vi "GDSString_XmlEnumToStringValue.vi"(0 "XmlEnumStringIn":string, 1 "EnumVariantIn(used if String is Empty)":variant, 5 "error in (no error)":errorcluster) -> (14 "EnumValueOut(string)":string, 15 "EnumItems(string)":string[](array[string]), 16 "EnumValueOut(uint16)":u16, 19 "error out":errorcluster)   [LabVIEW 2020]
doc: "Uses a flatten XML string of a Enum-type <B>\"XmlEnumStringIn\"</B> to find the acctually value of the enum.\nThis is normally used when a Enum has been flatten to a variant.\nIt could also take the enum variant as an input\nIt the Variant ENUM is of string type it will send it through without any errors"
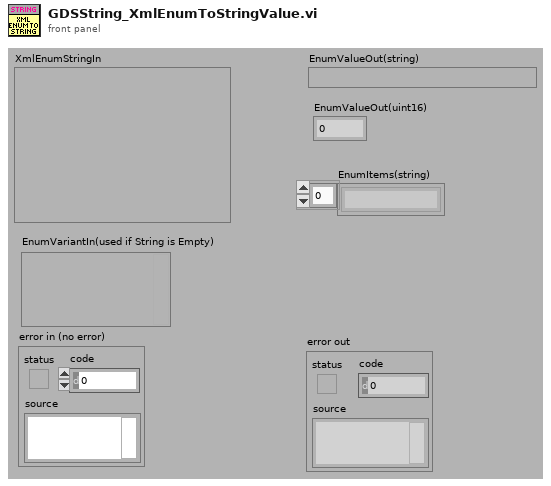
[diagram p1: front panel]
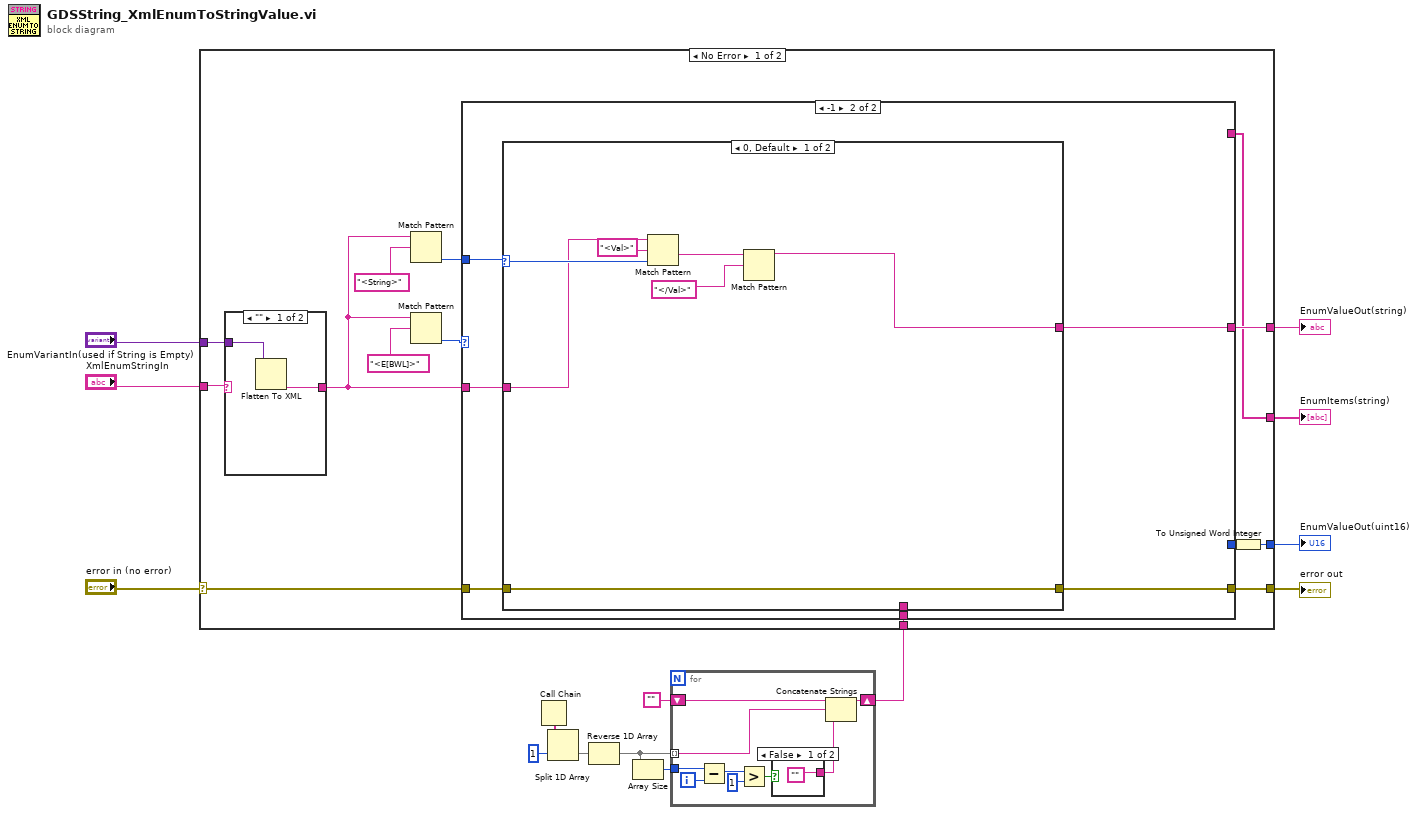
[diagram p0: block diagram]
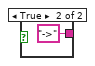
[diagram p2: hidden frame]
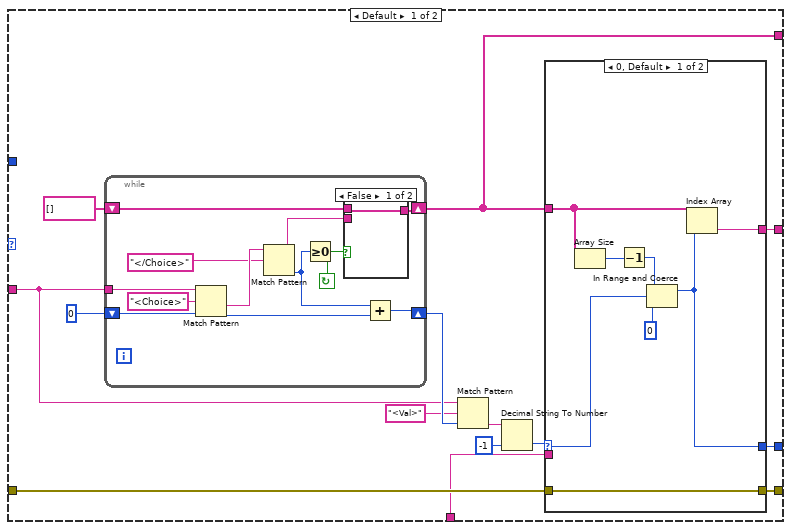
[diagram p4: hidden frame]
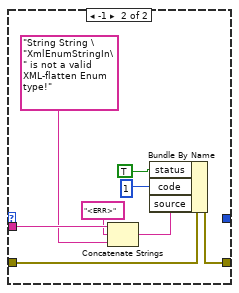
[diagram p5: hidden frame]
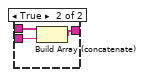
[diagram p6: hidden frame]
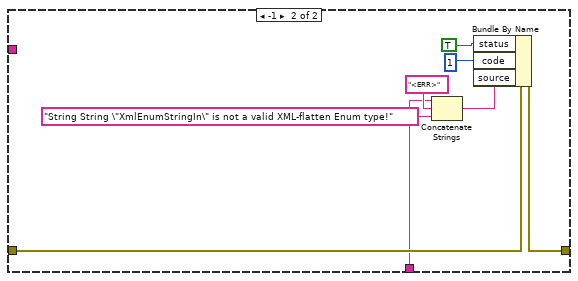
[diagram p7: hidden frame]
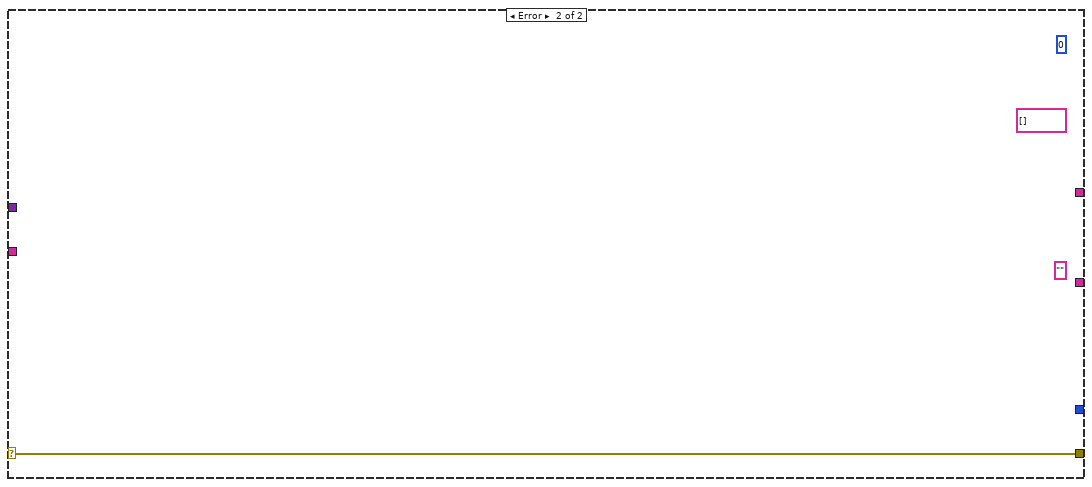
[diagram p8: hidden frame]
diagram:
  n1 = Call Chain() -> (call chain=w2:string[])
  n2 = Split 1D Array(array=w2, index=1) -> (second subarray=w4:string[])  [unwired: 1 out]
  n3 = Reverse 1D Array(array=w4) -> (reversed array=w7:string[])
  n4 = Array Size(array=w7) -> (size(s)=w5:i32)
  n5 = for {
    shift-right: [w15] -> w1
    shift-left: "" -> [w18]
    tunnel: w7 -> [w16] mode=indexing
    tunnel: w5 -> [w23]
    i -> [w22]
    n6 = Subtract(x=w23, y=w22) -> (x-y=w21:i32)
    n7 = Greater?(x=w21, y=1) -> (0:w19:bool)
    n8 = case shown="False" w19 {
      tunnel: ["" "->"] -> w17
      frame False {
      }
      frame True {
      }
    }
    n9 = Concatenate Strings(w18, w16, w17) -> (w15:string)
  }
  n10 = case shown="No Error" "error in (no error)" {
    selector: "error in (no error)" -> [w37 w110]
    tunnel: [w36 w110] -> w13
    tunnel: "XmlEnumStringIn" -> [w32 _]
    tunnel: [w35 _] -> w11
    tunnel: [w33 _] -> w10
    tunnel: "EnumVariantIn(used if String is Empty)" -> [w31 _]
    tunnel: [w27 _] -> w8
    tunnel: w1 -> [w26 _]
    frame No Error {
      n11 = case shown="\"\"" w32 {
        selector: w32 -> [_ w42]
        tunnel: [w40 w42] -> w29
        tunnel: w31 -> [w41 _]
        frame "" {
          n12 = Flatten To XML(6:w41) -> (2:w40:string)
        }
        frame Default {
        }
      }
      n13 = Match Pattern(string=w29, regular expression="<String>") -> (offset past match=w28:i32)  [unwired: 1 in, 3 out]
      n14 = Match Pattern(string=w29, regular expression="<E[BWL]>") -> (offset past match=w38:i32)  [unwired: 1 in, 3 out]
      n15 = case shown="-1" w38 {
        tunnel: w29 -> [w53 w91]
        tunnel: w37 -> [w48 w94]
        tunnel: [w47 w93] -> w36
        tunnel: [w46 w89] -> w35
        tunnel: [w45 _] -> w34
        tunnel: w28 -> [_ w92]
        tunnel: [w44 _] -> w27
        tunnel: w26 -> [w43 w90]
        frame Default {
          n16 = while {
            shift-left: 0 ("offset past match") -> [w82]
            shift-right: [w78] -> w54
            tunnel: w53 -> [w83]
            shift-right: [w74] -> w44
            shift-left: string[] [] -> [w75]
            stop <- w76 continue-if-true
            n17 = Match Pattern(string=w83, regular expression="<Choice>", offset (0)=w82) -> (after substring=w81:string, offset past match=w79:i32)  [unwired: 2 out]
            n18 = Match Pattern(string=w81, regular expression="</Choice>") -> (before substring=w73:string, offset past match=w77:i32)  [unwired: 1 in, 2 out]
            n19 = Greater Or Equal To 0?(x=w77) -> (x >= 0?=w76:bool)
            n20 = case shown="False" w76 {
              tunnel: w75 -> [w85 w88]
              tunnel: [w85 w87] -> w74
              tunnel: w73 -> [_ w86]
              frame False {
              }
              frame True {
                n21 = Build Array (concatenate)(w88, w86) -> (w87:string[])
              }
            }
            n22 = Add(x=w77, y=w79) -> (x+y=w78:i32)
          }
          n23 = Match Pattern(string=w53, regular expression="<Val>", offset (0)=w54) -> (after substring=w51:string)  [unwired: 3 out]
          n24 = Decimal String To Number(string=w51, default (0L)=-1 ("default (0 I32)")) -> (number=w49:i32)  [unwired: 1 in, 1 out]
          n25 = case shown="0, Default" w49 {
            selector: w49 -> [w59 _]
            tunnel: w48 -> [w64 w69]
            tunnel: [w64 w65] -> w47
            tunnel: w44 -> [w62 _]
            tunnel: [w63 _] -> w46
            tunnel: [w58 _] -> w45
            tunnel: w43 -> [_ w68]
            frame 0, Default {
              n26 = Array Size(array=w62) -> (size(s)=w61:i32)
              n27 = Decrement(x=w61) -> (x-1=w60:i32)
              n28 = In Range and Coerce(upper limit=w60, x=w59, lower limit=0) -> (coerced(x)=w58:i32)  [unwired: 1 out]
              n29 = Index Array(array=w62, index=w58) -> (element=w63:string)
            }
            frame -1 {
              n30 = Concatenate Strings(w68, "<ERR>" ("Substring"), "String String \"XmlEnumStringIn\" is not a valid XML-flatten Enum type!" ("source")) -> (w71:string)
              n31 = Bundle By Name(cluster=w69, "status"=TRUE ("Bundle Element"), "code"=1 ("code (5000)"), "source"=w71) -> (w65:errorcluster)
            }
          }
        }
        frame -1 {
          n32 = case shown="0, Default" w92 {
            selector: w92 -> [w100 _]
            tunnel: w94 -> [w96 w104]
            tunnel: [w96 w105] -> w93
            tunnel: [w97 _] -> w89
            tunnel: w91 -> [w95 _]
            tunnel: w90 -> [_ w102]
            frame 0, Default {
              n33 = Match Pattern(string=w95, regular expression="<Val>", offset (0)=w100) -> (after substring=w99:string)  [unwired: 3 out]
              n34 = Match Pattern(string=w99, regular expression="</Val>") -> (before substring=w97:string)  [unwired: 1 in, 3 out]
            }
            frame -1 {
              n35 = Concatenate Strings(w102, "<ERR>" ("Substring"), "String String \"XmlEnumStringIn\" is not a valid XML-flatten Enum type!" ("source")) -> (w108:string)
              n36 = Bundle By Name(cluster=w104, "status"=TRUE ("Bundle Element"), "code"=1 ("code (5000)"), "source"=w108) -> (w105:errorcluster)
            }
          }
        }
      }
      n37 = To Unsigned Word Integer(number=w34) -> (unsigned 16bit integer=w33:u16)
    }
    frame Error {
      (unwired) string[] []
      (unwired) 0
      (unwired) "" ("String in")
    }
  }
  "error out" <- w13
  "EnumValueOut(string)" <- w11
  "EnumValueOut(uint16)" <- w10
  "EnumItems(string)" <- w8
